vi "RWA control.vi"(3 "bytes to read":u32=5, 4 "VISA resource name (read)":refnum<visa-resource-name>="COM5", 5 "string to write":string="*IDN?\n", 6 "VISA resource name (write)":refnum<visa-resource-name>="COM4", 7 "flow control":u16(ring) items=["None"=0, "XON/XOFF"=1, "RTS/CTS"=2, "DTR/DSR"=4], 8 "stop bits":u16(ring)=10 items=["1.0"=10, "1.5"=15, "2.0"=20], 9 "parity (0:none)":u16(ring) items=["None", "Odd", "Even", "Mark", "Space"], 10 "data bits (8)":u16=8 min=5 max=8 step=1, 11 "baud rate (9600)":u32=115200) -> (0 "read string":string, 1 "bytes written":u32, 2 "bytes read":u32)   [LabVIEW 2012]
doc: "The Basic Serial Write and Read (2Port) example opens 2 VISA resources and configures one COM port to perform a write operation and the other COM port to perform a read operation. This VI will wait until the specified number of bytes (bytes to read) is received at the port or until a termination character is read.\n\nINSTRUCTIONS:\n1) Select the serial resource and configuration parameters (baud rate, data bits, parity, stop bits, flow control).\n2) Select the operations to be performed. \n3) Connect a null modem RS-232 or RS-485/422 cable between the 2 ports.\n4) Run the VI to see the \"read string\" match the \"string to write\".\n\nLike the Basic Serial Write and Read VI, this VI allows you perform diagnostic tests on your ports. You can use this VI to perform a wrapback test. Both serial ports must have the same basic configuration parameters. You can connect two of the ports using a null modem cable, which effectively connects one port's RX lines to the other port's TX lines. If you use a straight-through cable, one port's RX lines will be connected to the other port's RX lines, and you cannot communicate between the two ports. \n\nOn the block diagram, the VI calls the VISA Configure Serial Port VI twice, once for each of the two ports. This opens two separate VISA sessions. One VISA session performs the Write operation and the other performs the Read operation. Because two VISA sessions are opened, the VI includes two separate VISA Close functions."
uses:
  <vilib>/Instr/_visa.llb/VISA Configure Serial Port (Instr).vi
panel:
  # "On Windows/Linux, consider using the Instrument Driver Finder (Help>>Find Instrument Drivers) to search for an instrument driver for your instrument."
  # "Select the appropriate VISA Resource Names for the two ports (read and write). Also set the port configuration parameters on the front panel (baud rate, data bits, parity, stop bits and flow control).   Before executing the VI, connect a null modem  cable between the two ports you would like to work with."
  # "For additional information select File >> VI Properties >> Documentation"
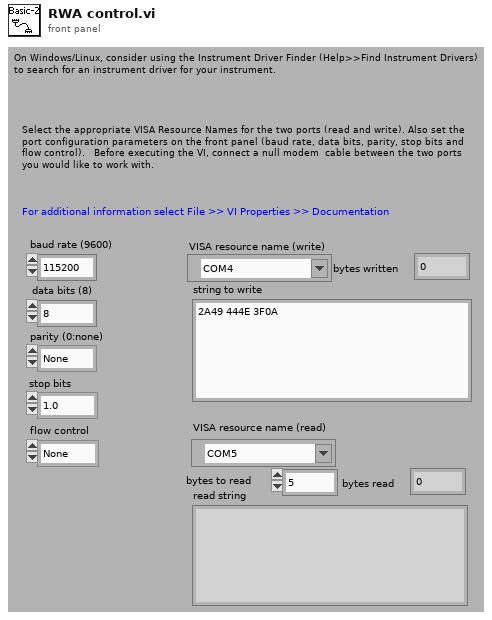
[diagram p1: front panel]
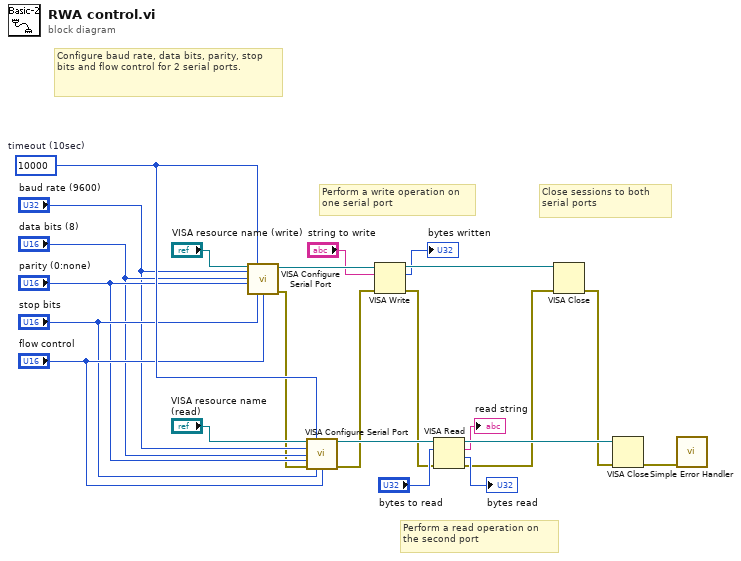
[diagram p0: block diagram]
diagram:
  w13 = u32 10000  # timeout (10sec)
  # "Close sessions to both serial ports"
  # "Perform a write operation on one serial port"
  # "Perform a read operation on the second port"
  # "Configure baud rate, data bits, parity, stop bits and flow control for 2 serial ports."
  n1 = call-poly "VISA Configure Serial Port"("VISA resource name"="VISA resource name (write)", "timeout (10sec)"=w13, "baud rate (9600)"="baud rate (9600)", "data bits (8)"="data bits (8)", "parity (0:none)"="parity (0:none)", "stop bits (10: 1 bit)"="stop bits", "flow control (0:none)"="flow control") -> ("VISA resource name out"=w22:refnum<visa-resource-name>, "error out"=w6:errorcluster)  [unwired: 2 in, 5 out]
  n2 = call-poly "VISA Configure Serial Port"("VISA resource name"="VISA resource name (read)", "timeout (10sec)"=w13, "baud rate (9600)"="baud rate (9600)", "data bits (8)"="data bits (8)", "parity (0:none)"="parity (0:none)", "error in (no error)"=w6, "stop bits (10: 1 bit)"="stop bits", "flow control (0:none)"="flow control") -> ("VISA resource name out"=w20:refnum<visa-resource-name>, "error out"=w5:errorcluster)  [unwired: 2 in, 4 out]
  n3 = VISA Write(VISA resource name=w22, write buffer="string to write", error in (no error)=w5) -> (VISA resource name out=w21:refnum<visa-resource-name>, return count=→"bytes written":u32, error out=w4:errorcluster)
  n4 = VISA Read(VISA resource name=w20, byte count="bytes to read", error in (no error)=w4) -> (VISA resource name out=w19:refnum<visa-resource-name>, read buffer=→"read string":string, return count=→"bytes read":u32, error out=w3:errorcluster)
  n5 = VISA Close(VISA resource name=w21, error in (no error)=w3) -> (error out=w2:errorcluster)
  n6 = VISA Close(VISA resource name=w19, error in (no error)=w2) -> (error out=w1:errorcluster)
  n7 = call <vilib>:"Simple Error Handler.vi"("error in (no error)"=w1) -> ()  [unwired: 1 in, 8 out]
